vi "DEMO.vi"() -> ()   [LabVIEW 2011]
panel:
  in  "Select Receiver":string(combo)
  in  "停止":bool
  out "Message 2":string
  out "Sender 2":string
  out "Receiver 2":string
  out "Receiver":string
  out "Sender":string
  out "Message":string
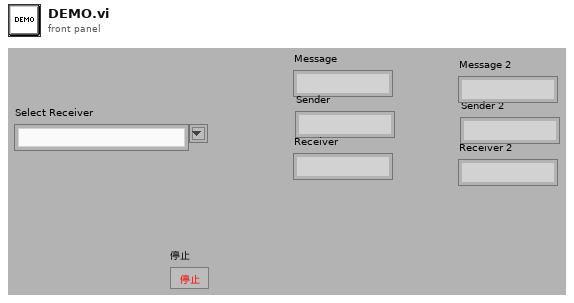
[diagram p1: front panel]
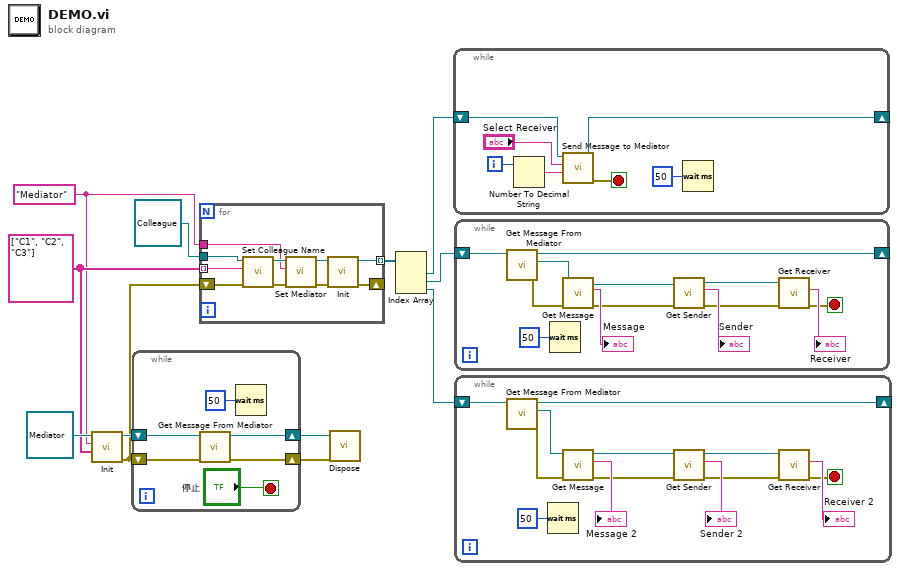
[diagram p0: block diagram]
diagram:
  w11 = string[] ["C1", "C2", "C3"] ("Colleague Names")
  w9 = "Mediator" ("Mediator Name")
  n1 = call "Init.vi"("Colleague Names"=w11, "Mediator Name"=w9, "Mediator 输入"=refnum<class "Mediator.lvclass"> refnum ("Mediator.lvclass")) -> ("error out"=w7:errorcluster, "Mediator 输出"=w8:refnum<class "Mediator.lvclass">)  [unwired: 7 in]
  n2 = while {
    shift-right: [w16] -> w2
    shift-left: w8 -> [w17]
    shift-right: [w14] -> w1
    shift-left: w7 -> [w15]
    stop <- "停止" stop-if-true
    n3 = call "Get Message From Mediator.vi"("error in (no error)"=w15, "Mediator 输入"=w17) -> ("error out"=w14:errorcluster, "Mediator 输出"=w16:refnum<class "Mediator.lvclass">)  [unwired: 8 in]
    n4 = Wait (ms)(milliseconds to wait=u32 50 ("等待时间（毫秒）")) -> ()  [unwired: 1 out]
  }
  n5 = for {
    tunnel: w11 -> [w27] mode=indexing
    tunnel: refnum<class "Colleague.lvclass"> refnum ("Colleague.lvclass") -> [w28]
    shift-right: [w21] -> _
    shift-left: w7 -> [w26]
    tunnel: [w20] -> w6 mode=indexing
    tunnel: w9 -> [w19]
    n6 = call "Set Colleague Name.vi"("error in (no error)"=w26, "同事名称"=w27, "同事（抽象）输入"=w28) -> ("error out"=w25:errorcluster, "同事（抽象）输出"=w23:refnum<class "Colleague.lvclass">)  [unwired: 7 in]
    n7 = call "Set Mediator.vi"("error in (no error)"=w25, "Mediator"=w19, "Colleague输入"=w23) -> ("error out"=w24:errorcluster, "Colleague输出"=w22:refnum<class "Colleague.lvclass">)  [unwired: 7 in]
    n8 = call "Init.vi"("error in (no error)"=w24, "同事（抽象） 输入"=w22) -> ("error out"=w21:errorcluster, "同事（抽象） 输出"=w20:refnum<class "Colleague.lvclass">)  [unwired: 8 in]
  }
  n9 = call "Dispose.vi"("error in (no error)"=w1, "Mediator 输入"=w2) -> ()  [unwired: 8 in, 2 out]
  n10 = Index Array(array=w6) -> (element #1=w5:refnum<class "Colleague.lvclass">, element #2=w4:refnum<class "Colleague.lvclass">, element #3=w3:refnum<class "Colleague.lvclass">)  [unwired: 3 in]
  n11 = while {
    shift-right: [w34] -> _
    shift-left: w5 -> [w35]
    i -> [w31]
    stop <- w32 stop-if-true
    n12 = Number To Decimal String(number=w31) -> (decimal integer string=w30:string)  [unwired: 1 in]
    n13 = call "Send Message to Mediator.vi"("Message"=w30, "Receiver"="Select Receiver", "Colleague 输入"=w35) -> ("error out"=w32:errorcluster, "Colleague 输出"=w34:refnum<class "Colleague.lvclass">)  [unwired: 7 in]
    n14 = Wait (ms)(milliseconds to wait=u32 50 ("等待时间（毫秒）")) -> ()  [unwired: 1 out]
  }
  n15 = while {
    shift-right: [w47] -> _
    shift-left: w4 -> [w48]
    stop <- w39 stop-if-true
    n16 = call "Get Message From Mediator.vi"("Colleague 输入"=w48) -> ("error out"=w45:errorcluster, "Message.lvclass"=w46:refnum<class "Message.lvclass">, "Colleague 输出"=w47:refnum<class "Colleague.lvclass">)  [unwired: 8 in]
    n17 = Wait (ms)(milliseconds to wait=u32 50 ("等待时间（毫秒）")) -> ()  [unwired: 1 out]
    n18 = call "Get Message.vi"("error in (no error)"=w45, "Message输入"=w46) -> ("error out"=w38:errorcluster, "Message"=→"Message":string, "Message输出"=w43:refnum<class "Message.lvclass">)  [unwired: 7 in]
    n19 = call "Get Sender.vi"("error in (no error)"=w38, "Message输入"=w43) -> ("error out"=w37:errorcluster, "Sender"=→"Sender":string, "Message输出"=w41:refnum<class "Message.lvclass">)  [unwired: 7 in]
    n20 = call "Get Receiver.vi"("error in (no error)"=w37, "Message输入"=w41) -> ("error out"=w39:errorcluster, "Receiver"=→"Receiver":string)  [unwired: 7 in, 1 out]
  }
  n21 = while {
    shift-right: [w60] -> _
    shift-left: w3 -> [w61]
    stop <- w51 stop-if-true
    n22 = call "Get Message From Mediator.vi"("Colleague 输入"=w61) -> ("error out"=w58:errorcluster, "Message.lvclass"=w59:refnum<class "Message.lvclass">, "Colleague 输出"=w60:refnum<class "Colleague.lvclass">)  [unwired: 8 in]
    n23 = Wait (ms)(milliseconds to wait=u32 50 ("等待时间（毫秒）")) -> ()  [unwired: 1 out]
    n24 = call "Get Message.vi"("error in (no error)"=w58, "Message输入"=w59) -> ("error out"=w50:errorcluster, "Message"=→"Message 2":string, "Message输出"=w55:refnum<class "Message.lvclass">)  [unwired: 7 in]
    n25 = call "Get Sender.vi"("error in (no error)"=w50, "Message输入"=w55) -> ("error out"=w49:errorcluster, "Sender"=→"Sender 2":string, "Message输出"=w53:refnum<class "Message.lvclass">)  [unwired: 7 in]
    n26 = call "Get Receiver.vi"("error in (no error)"=w49, "Message输入"=w53) -> ("error out"=w51:errorcluster, "Receiver"=→"Receiver 2":string)  [unwired: 7 in, 1 out]
  }
